vi "AMZ_S3_APIHLP_Parse ListBucketResult.vi"(8 "error in (no error)":errorcluster, 10 "Response body":string) -> (0 "error out":errorcluster, 3 "ListBucketResult":T1)   [LabVIEW 2015, in "LV Interface for Amazon S3.lvlib"]
doc: "Parse out the Results from the Response body of a List bucket request."
uses:
  LV Interface for Amazon S3.lvlib
  Typedefs/AMZ_S3_API_ListBucketResult.ctl
  Typedefs/AMZ_S3_API_ListBucketResult Content.ctl
  Typedefs/AMZ_S3_Storage Class.ctl
  Typedefs/AMZ_S3_API_Owner.ctl
  Typedefs/AMZ_S3_API_ListBucketResult CommonPrefix.ctl
  XML Parser/XML Parser.lvlib
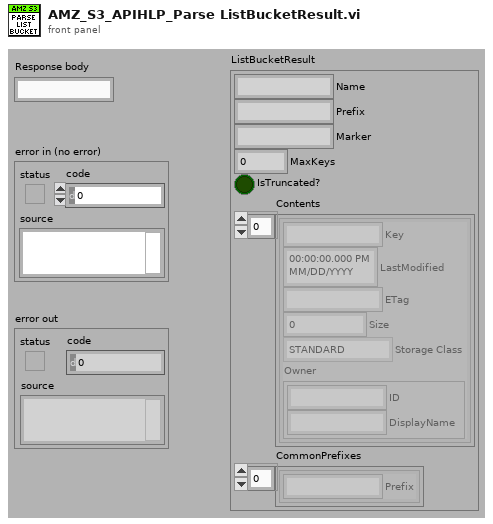
[diagram p1: front panel]
types:
  T1 = typedef "LV Interface for Amazon S3.lvlib/AMZ_S3_API_ListBucketResult.ctl" = cluster{"Name":string, "Prefix":string, "Marker":string, "MaxKeys":u16, "IsTruncated?":bool, "Contents":T2[], "CommonPrefixes":T5[]}
  T2 = typedef "LV Interface for Amazon S3.lvlib/AMZ_S3_API_ListBucketResult Content.ctl" = cluster{"Key":string, "LastModified":timestamp, "ETag":string, "Size":u64, "Storage Class":T3, "Owner":T4}
  T3 = typedef "LV Interface for Amazon S3.lvlib/AMZ_S3_Storage Class.ctl" = enum16{"STANDARD", "REDUCED_REDUNDANCY"}
  T4 = typedef "LV Interface for Amazon S3.lvlib/AMZ_S3_API_Owner.ctl" = cluster{"ID":string, "DisplayName":string}
  T5 = typedef "LV Interface for Amazon S3.lvlib/AMZ_S3_API_ListBucketResult CommonPrefix.ctl" = cluster{"Prefix":string}
  T6 = cluster{"[0]":string, "[1]":string, "[2]":string, "[3]":string, "[4]":string}
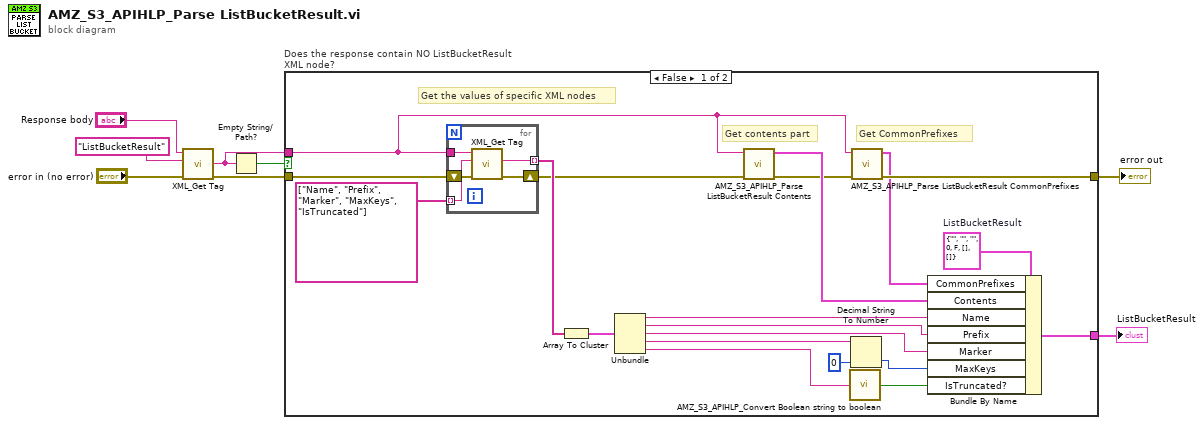
[diagram p0: block diagram]
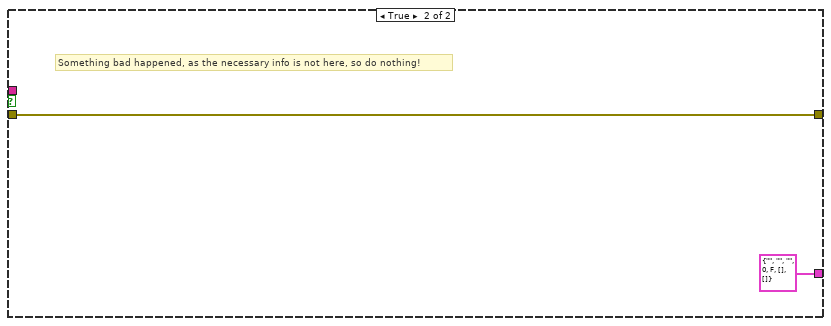
[diagram p2: hidden frame]
diagram:
  n1 = call "XML_Get Tag.vi"("error in (no error)"="error in (no error)", "Tag name"="ListBucketResult", "XML String in"="Response body") -> ("error out"=w2:errorcluster, "Tag value"=w1:string)  [unwired: 4 in, 3 out]
  n2 = Empty String/Path?(string/path=w1) -> (empty?=w3:bool)
  n3 = case "Does the response contain NO ListBucketResult XML node?" shown="False" w3 {
    tunnel: w1 -> [w9 _]
    tunnel: w2 -> [w20 w35]
    tunnel: [w27 T1 {"Name"="", "Prefix"="", "Marker"="", "MaxKeys"=0, "IsTruncated?"=FALSE, "Contents"=[], "CommonPrefixes"=[]} ("ListBucketResult")] -> w8
    tunnel: [w24 w35] -> w7
    frame False {
      w22 = T1 {"Name"="", "Prefix"="", "Marker"="", "MaxKeys"=0, "IsTruncated?"=FALSE, "Contents"=[], "CommonPrefixes"=[]}  # ListBucketResult
      # "Get the values of specific XML nodes"
      # "Get CommonPrefixes"
      # "Get contents part"
      n4 = for {
        tunnel: string[] ["Name", "Prefix", "Marker", "MaxKeys", "IsTruncated"] -> [w32] mode=indexing
        tunnel: w9 -> [w31]
        tunnel: [w30] -> w19 mode=indexing
        shift-right: [w29] -> w10
        shift-left: w20 -> [w33]
        n5 = call "XML_Get Tag.vi"("error in (no error)"=w33, "Tag name"=w32, "XML String in"=w31) -> ("error out"=w29:errorcluster, "Tag value"=w30:string)  [unwired: 4 in, 3 out]
      }
      n6 = Array To Cluster(array=w19) -> (cluster=w18:T6)
      n7 = Unbundle(w18) -> ("[0]"=w17:string, "[1]"=w16:string, "[2]"=w15:string, "[3]"=w14:string, "[4]"=w12:string)
      n8 = call "AMZ_S3_APIHLP_Parse ListBucketResult Contents.vi"("error in (no error)"=w10, "Response body"=w9) -> ("error out"=w25:errorcluster, "Contents"=w26:T2[])  [unwired: 8 in]
      n9 = call "AMZ_S3_APIHLP_Convert Boolean string to boolean.vi"("Boolean string in"=w12) -> ("Boolean out"=w11:bool)  [unwired: 4 in]
      n10 = Decimal String To Number(string=w14, default (0L)=u16 0) -> (number=w13:u16)  [unwired: 1 in, 1 out]
      n11 = call "AMZ_S3_APIHLP_Parse ListBucketResult CommonPrefixes.vi"("error in (no error)"=w25, "Response body"=w9) -> ("error out"=w24:errorcluster, "CommonPrefixes"=w23:T5[])  [unwired: 8 in]
      n12 = Bundle By Name(cluster=w22, "CommonPrefixes"=w23, "Contents"=w26, "Name"=w17, "Prefix"=w16, "Marker"=w15, "MaxKeys"=w13, "IsTruncated?"=w11) -> (w27:T1)
    }
    frame True {
      # "Something bad happened, as the necessary info is not here, so do nothing!"
    }
  }
  "ListBucketResult" <- w8
  "error out" <- w7
